vi "SQL Query.vi"(8 "error in (no error)":errorcluster, 10 "SQL Server Info":T2={"Port"=3306, "IP Address"="192.168.10.63", "Authentication"={"User"="loasis", "Password"="dat+l0sim", "Database"="loasis"}}, 11 "Query":string="SELECT devicetype_variable.name, devicetype_variable.defaultvalue, devicetype_variable.min, devicetype_variable.max, devicetype_variable.stepsize, devicetype_variable.units, devicetype_variable.variabletype\nFROM devicetype_variable\nWHERE (NOT EXISTS\n  (select *\n    from variable\n    where devicetype_variable.id = variable.devicetype_variable_id)) AND\n  (devicetype_variable.devicetype = (SELECT devicetype FROM device WHERE name='TREX Mode Imager'))\n  UNION\n  SELECT variable.name, variable.defaultvalue, variable.min, variable.max, variable.stepsize, variable.units, variable.variabletype FROM variable WHERE device='TREX Mode Imager';") -> (0 "error out":errorcluster, 3 "data":string[][](array[string]))   [LabVIEW 2011]
uses:
  shared programs/MySQL/database configuration.ctl
  shared programs/MySQL/typedefs/mysql_authentication.ctl
panel:
  in  "Tab Control":T1(tab)=enum."internal"
  out "Return Data":variant[][](array[variant])=[[variant(string "Trigger"), variant(string "off"), variant(string ""), variant(string ""), variant(string ""), variant(string "choice"), variant], [variant(string "Local Save Path"), variant(string "c:\\temp"), variant(string ""), variant(string ""), variant(string ""), variant(string "string"), variant], [variant(string "Image"), variant(string ""), variant(string ""), variant(string ""), variant(string ""), variant(string "image"), variant], [variant(string "Exposure"), variant(string "0.11"), variant(string "0"), variant(string "1"), variant(string "0.1"), variant(string "s"), variant(string "numeric")]]
  # "SELECT * FROM variable JOIN devicetype_variable ON variable.devicetype_variable_id=devicetype_variable.id;"
  # "Get name column from device table\nSELECT name FROM device;\ni.e. gets all devices"
  # "Get all data from variable table\nSELECT * FROM variable;\nNote that only variables overidden from devicetype_variable will be got from this call. To get all variables you need to look at both\nvariable and devicetype_variable tables"
  # "Get all setable variables of a device called TREX Mode Imager\nSELECT devicetype_variable.name, devicetype_variable.defaultvalue, devicetype_variable.min, devicetype_variable.max, devicetype_variable.stepsize, devicetype_variable.units, devicetype_variable.variabletype\nFROM devicetype_variable\nWHERE (NOT EXISTS\n  (select *\n    from variable\n    where devicetype_variable.id = variable.devicetype_variable_id)) AND\n  (devicetype_variable.devicetype = (SELECT devicetype FROM device WHERE name='TREX Mode Imager'))  AND devicetype_variable.set='yes'\n  UNION\n  SELECT variable.name, variable.defaultvalue, variable.min, variable.max, variable.stepsize, variable.units, variable.variabletype FROM variable WHERE device='TREX Mode Imager' AND variable.set='yes';"
  # "Get all variables of a device called TREX Mode Imager\nSELECT devicetype_variable.name, devicetype_variable.defaultvalue, devicetype_variable.min, devicetype_variable.max, devicetype_variable.stepsize, devicetype_variable.units, devicetype_variable.variabletype\nFROM devicetype_variable\nWHERE (NOT EXISTS\n  (select *\n    from variable\n    where devicetype_variable.id = variable.devicetype_variable_id)) AND\n  (devicetype_variable.devicetype = (SELECT devicetype FROM device WHERE name='TREX Mode Imager'))\n  UNION\n  SELECT variable.name, variable.defaultvalue, variable.min, variable.max, variable.stepsize, variable.units, variable.variabletype FROM variable WHERE device='TREX Mode Imager';"
  # "Get basic properties of a device\nSELECT * FROM device WHERE device.name='TREX Mode Imager';\n\nOR you can specify columns like this\n\nSELECT device.devicetype, device.ipaddress, device.commport, device.location, device.class\nFROM device WHERE device.name='TREX Mode Imager';"
  # "Get network communication port of a device\nSELECT device.commport\nFROM device WHERE device.name='TREX Mode Imager';"
  # "Get MultiCast IP address of selected experiment\nSELECT expt.MultiCastIP FROM expt WHERE expt.name='TREX low power';"
  # "SELECT p1.default, p2.default\n FROM cam1 AS p1 INNER JOIN cam2 AS p2 \nON p1.variable = p1.variable  AND  p1.variable='IP' AND  p2.variable='IP';"
  # "CREATE DEVICE CAM"
  # "UPDATE `cam1`.`var2` SET `t1`=4 WHERE `idvar2`='1';"
  # "CREATE  TABLE `cam1`.`var2` (\n\n  `idvar2` INT NOT NULL ,\n\n  `t1` INT NULL ,\n\n  `t2` YEAR NULL ,\n\n  `t3` TINYINT(1)  NULL ,\n\n  PRIMARY KEY (`idvar2`) );"
  # "CREATE  TABLE `devices`.`Cam2` (\n\n  `idCam2` INT NOT NULL ,\n\n  `variable` VARCHAR(45) NULL ,\n\n  `data type` VARCHAR(45) NULL ,\n\n  `default` VARCHAR(45) NULL ,\n\n  `min` VARCHAR(45) NULL ,\n\n  `max` VARCHAR(45) NULL ,\n\n  `access (read)` VARCHAR(45) NULL ,\n\n  `access(write)` VARCHAR(45) NULL ,\n\n  PRIMARY KEY (`idCam2`) );"
  # "SELECT * FROM port WHERE Device = 'Cam2';"
  # "SELECT p1.IP, p2.UDPport\n FROM ip AS p1 INNER JOIN port AS p2 \nON p1.Device = p1.Device AND p1.Device='Cam1' AND p2.Device='Cam1';"
  # "SELECT * FROM Cam1 WHERE accessWrite = 'false';"
  # "SELECT name  FROM variable WHERE device_name='TREX Mode Imager';"
  # "SELECT * FROM ip WHERE Device = 'Cam2';"
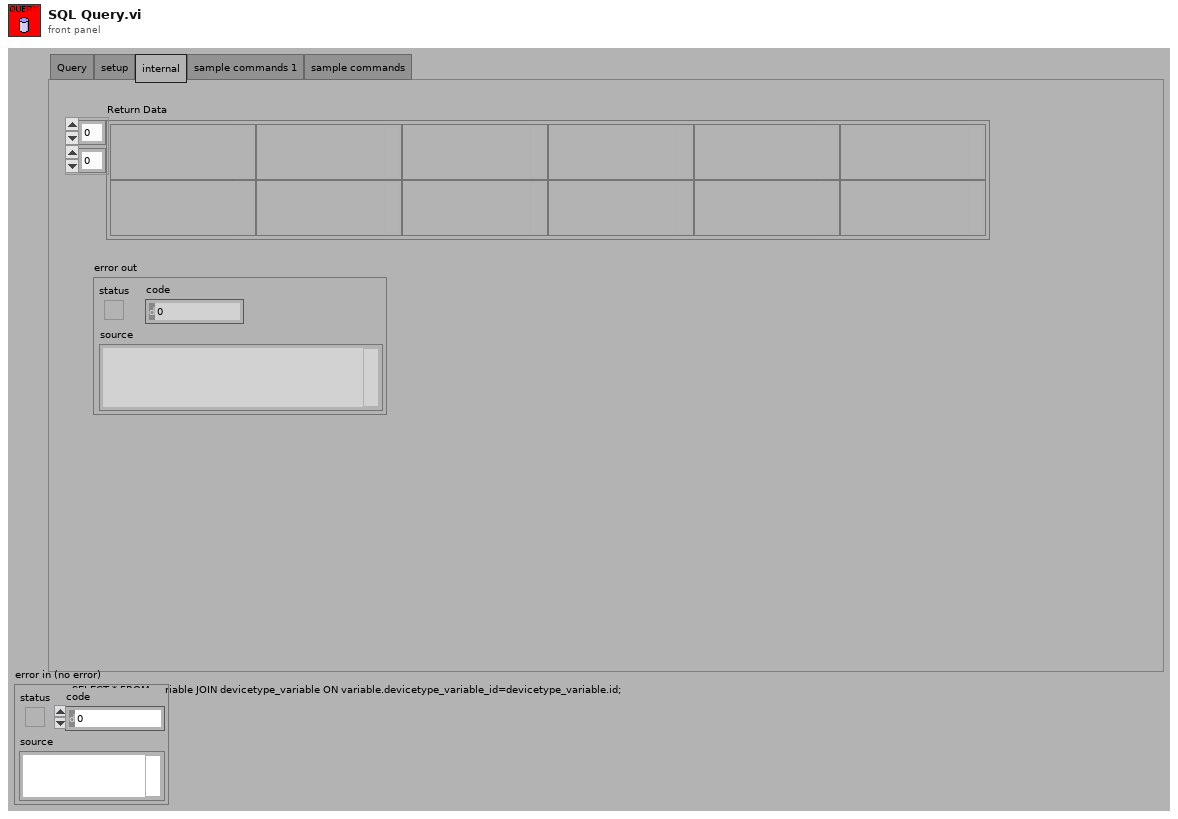
[diagram p1: front panel]
types:
  T1 = enum32{"Query", "setup", "internal", "sample commands 1", "sample commands"}
  T2 = typedef "database configuration.ctl" = cluster{"Port":u16, "IP Address":string, "Authentication":T3}
  T3 = typedef "mysql_authentication.ctl" = cluster{"User":string, "Password":string, "Database":string}
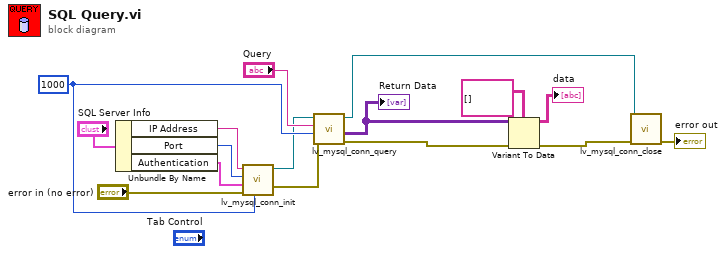
[diagram p0: block diagram]
diagram:
  w13 = 1000 ("timeout ms (60000)")
  n1 = Unbundle By Name("SQL Server Info") -> ("IP Address"=w6:string, "Port"=w5:u16, "Authentication"=w4:T3)
  n2 = call "lv_mysql_conn_init.vi"("timeout ms (5000)"=w13, "error in (no error)"="error in (no error)", "Authentication"=w4, "Port"=w5, "IP Address"=w6) -> ("error out"=w2:errorcluster, "connection ID out"=w8:refnum<k5>)  [unwired: 5 in]
  n3 = call "lv_mysql_conn_query.vi"("error in (no error)"=w2, "timeout ms (5000)"=w13, "Query"="Query", "connection ID"=w8) -> ("error out"=w12:errorcluster, "Return Data"=w11:variant[][], "connection ID out"=w15:refnum<k5>)  [unwired: 4 in, 1 out]
  "Return Data" <- w11
  n4 = Variant To Data(error in=w12, type=string[][] [], Variant=w11) -> (data=→"data":string[][], error out=w1:errorcluster)
  n5 = call "lv_mysql_conn_close.vi"("error in (no error)"=w1, "connection ID"=w15) -> ("error out"=→"error out":errorcluster)  [unwired: 9 in]
